vi "Facade.vi"(0 "Data In":T4, 2 "Display State In":T2, 3 "Container State":T3) -> (6 "Data Out":T4, 7 "Display State Out":T2, 8 "Action":T1)   [LabVIEW 2020, in "WebView2 XControl.lvlib" / "WebView2 Control.xctl"]
uses:
  WebView2 Control.xctl
  Data.ctl
  <vilib>/_xctls/Container State.ctl
  State.ctl
  Webview2 Lib/WebView2 Control Object/WebView2 Control.lvclass
  <vilib>/_xctls/Action.ctl
  Webview2 Lib/WebView2 Control Object/WebView2 Control.lvclass/WebView2 Control.ctl
  Webview2 Lib/WebView2 Control Object/Write Start URL.vi
  Webview2 Lib/WebView2 Control Object/Write URL.vi
  <vilib>/_xctls/XControlSupport.lvlib
  C:/Users/Simon/Documents/GitHub/LV-WebView2/Source/Libs/Microsoft.Web.WebView2.WinForms.dll
  Libs/Microsoft.Web.WebView2.WinForms.dll
panel:
  in  "WebView2":refnum<k24>(container)
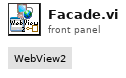
[diagram p1: front panel]
types:
  T1 = typedef "XControlSupport.lvlib/Action.ctl" = cluster{"Data Changed?":bool, "State Changed?":bool, "Action Name":string}
  T2 = typedef "WebView2 XControl.lvlib/WebView2 Control.xctl/State.ctl" = cluster{"Control Object Ref":refnum<data-value>}
  T3 = typedef "XControlSupport.lvlib/Container State.ctl" = cluster{"Indicator?":bool, "Run Mode?":bool, " Refnum":refnum<vi>}
  T4 = typedef "WebView2 XControl.lvlib/WebView2 Control.xctl/Data.ctl" = string
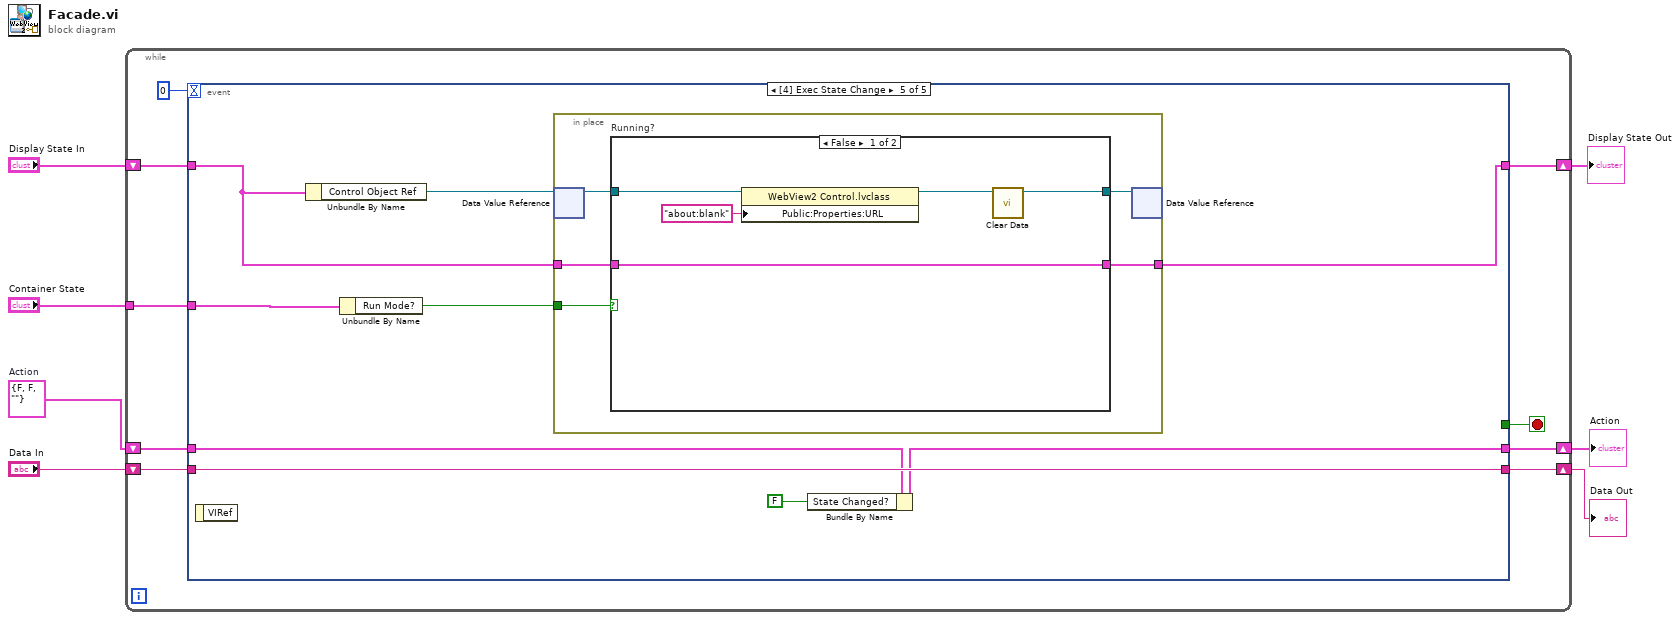
[diagram p0: block diagram]
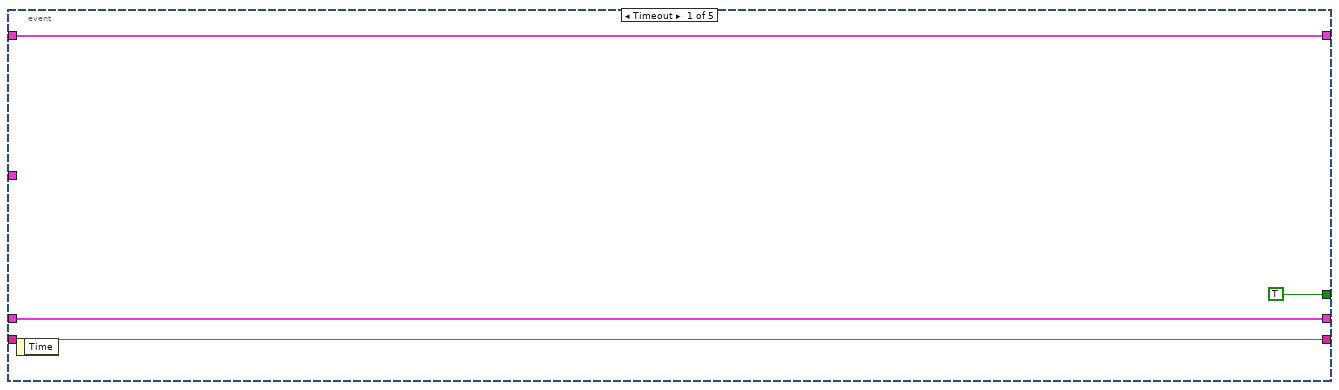
[diagram p2: hidden frame]
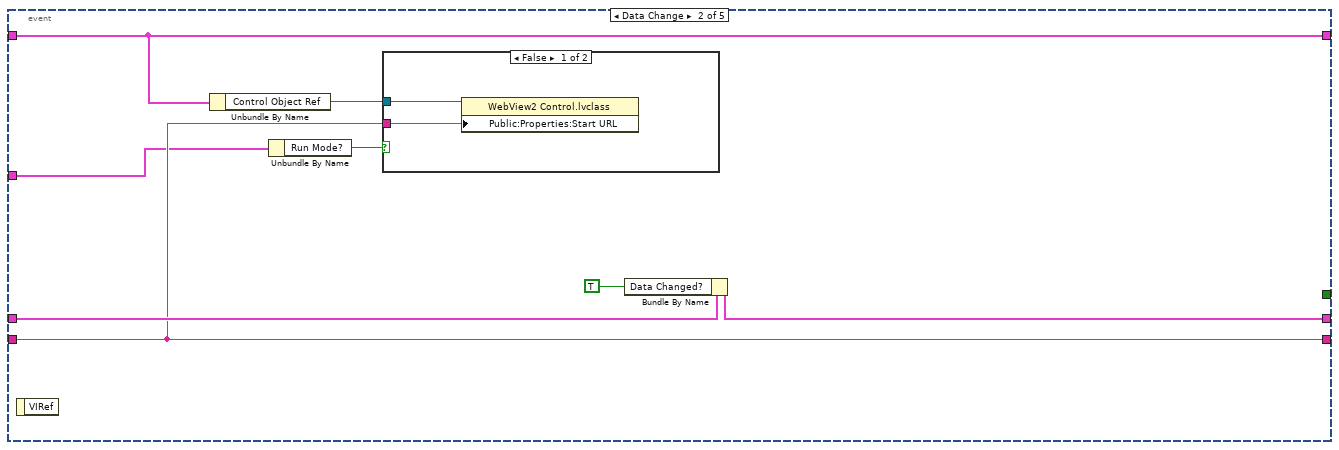
[diagram p3: hidden frame]
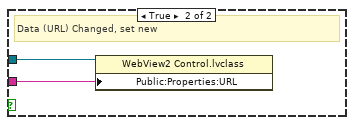
[diagram p4: hidden frame]
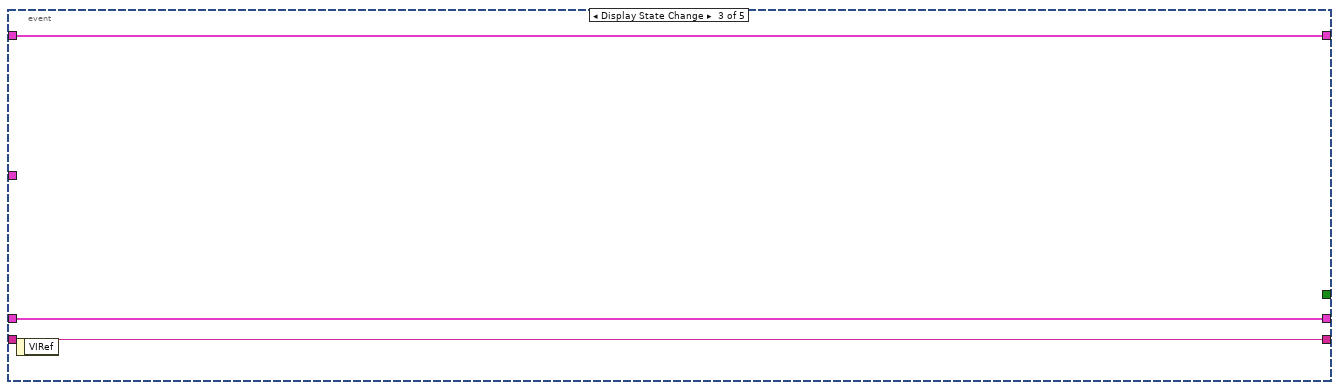
[diagram p5: hidden frame]
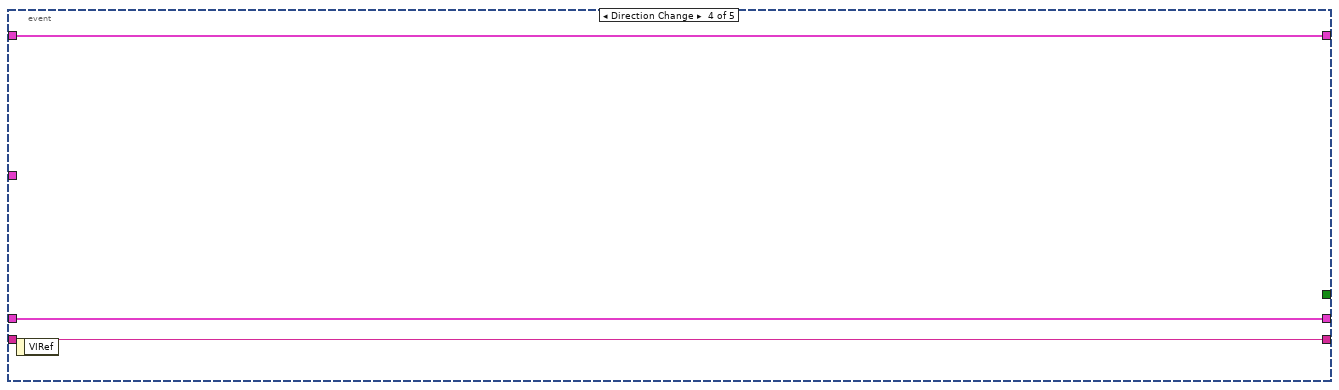
[diagram p6: hidden frame]
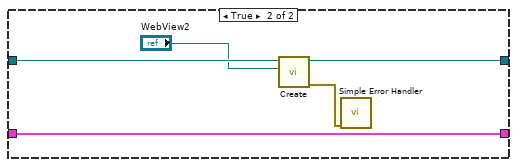
[diagram p7: hidden frame]
diagram:
  w2 = T1 {"Data Changed?"=FALSE, "State Changed?"=FALSE, "Action Name"=""}  # Action
  n1 = while {
    tunnel: "Container State" -> [w11]
    shift-right: [w16] -> w6
    shift-left: "Data In" -> [w15]
    shift-right: [w13] -> w3
    shift-left: w2 -> [w12]
    shift-right: [w14] -> w4
    shift-left: "Display State In" -> [w10]
    stop <- w8 stop-if-true
    n2 = event shown="[4] Exec State Change" {
      selector: _ -> [_ _ _ _ _]
      dyn-events: _ -> [_ _ _ _ _]
      timeout: 0 -> [_ _ _ _ _]
      tunnel: w10 -> [w18 w24 w35 w38 w42]
      tunnel: [w18 w24 w35 w38 w41] -> w14
      tunnel: [TRUE _ _ _ _] -> w8
      tunnel: w11 -> [_ w25 _ _ w47]
      tunnel: w15 -> [w17 w27 w34 w37 w46]
      tunnel: [w17 w27 w34 w37 w46] -> w16
      tunnel: [w19 w22 w33 w36 w40] -> w13
      tunnel: w12 -> [w19 w28 w33 w36 w45]
      event Timeout {
        n3 = event-data() -> ()  [unwired: 1 in, 1 out]
      }
      event Data Change {
        n4 = event-data() -> ()  [unwired: 1 in, 1 out]
        n5 = Unbundle By Name(w24) -> ("Control Object Ref"=w23:refnum<data-value>)
        n6 = Unbundle By Name(w25) -> ("Run Mode?"=w26:bool)
        n7 = case shown="False" w26 {
          tunnel: w27 -> [w29 w31]
          tunnel: w23 -> [w30 w32]
          frame False {
            n8 = property class="WebView2 Control.lvclass"(reference=w30, "Public:Properties:Start URL"=w29) -> ()  [unwired: 1 in, 2 out]
          }
          frame True {
            # "Data (URL) Changed, set new"
            n9 = property class="WebView2 Control.lvclass"(reference=w32, "Public:Properties:URL"=w31) -> ()  [unwired: 1 in, 2 out]
          }
        }
        n10 = Bundle By Name(cluster=w28, "Data Changed?"=TRUE) -> (w22:T1)
      }
      event Display State Change {
        n11 = event-data() -> ()  [unwired: 1 in, 1 out]
      }
      event Direction Change {
        n12 = event-data() -> ()  [unwired: 1 in, 1 out]
      }
      event Exec State Change {
        n13 = event-data() -> ()  [unwired: 1 in, 1 out]
        n14 = Unbundle By Name(w42) -> ("Control Object Ref"=w43:refnum<data-value>)
        n15 = Unbundle By Name(w47) -> ("Run Mode?"=w44:bool)
        n16 = in-place {
          in-place-border: w44 -> [w52]
          in-place-border: w42 -> [w49]
          in-place-border: [w48] -> w41
          n17 = in-place-dvr #1(w43) -> (w51:refnum<class "WebView2 Control.lvclass">)  [unwired: 1 out]
          n18 = case "Running?" shown="False" w52 {
            tunnel: w51 -> [w57 w60]
            tunnel: [w53 w62] -> w50
            tunnel: w49 -> [w55 w61]
            tunnel: [w55 w61] -> w48
            frame False {
              n19 = property class="WebView2 Control.lvclass"(reference=w57, "Public:Properties:URL"="about:blank" ("Site:URL")) -> (reference out=w56:refnum<class "WebView2 Control.lvclass">)  [unwired: 1 in, 1 out]
              n20 = call "Clear Data.vi"("WebView2 Control in"=w56) -> ("WebView2 Control out"=w53:refnum<class "WebView2 Control.lvclass">)  [unwired: 9 in, 1 out]
            }
            frame True {
              n21 = call "Create.vi"("WebView2 Control"="WebView2", "Type"=w60) -> ("error out"=w59:errorcluster, "WebView2 Control out"=w62:refnum<class "WebView2 Control.lvclass">)  [unwired: 8 in]
              n22 = call <vilib>:"Simple Error Handler.vi"("error in (no error)"=w59) -> ()  [unwired: 4 in, 5 out]
            }
          }
          n23 = in-place-dvr #1(w50) -> ()  [unwired: 2 out]
        }
        n24 = Bundle By Name(cluster=w45, "State Changed?"=FALSE) -> (w40:T1)
      }
    }
  }
  "Display State Out" <- w4
  "Data Out" <- w6
  "Action" <- w3
